vi "N Closest Point.vi"(6 "Index to ignore Array":i32[](array[numeric]), 8 "line index":i32, 9 "Y in":dbl=359.5 format="%#_13g", 10 "X in":dbl=18.050867335505 format="%#_13g", 11 "All Lines":T1) -> (0 "Index on Line":i32, 3 "Array size":i32)   [LabVIEW 2014]
uses:
  Libraries/Map Data Folder/All-Lines.ctl
  Libraries/Map Data Folder/LineCluster.ctl
  Libraries/Map Data Folder/LineConnection.ctl
  Libraries/Map Data Folder/Map Data.lvlib
panel:
  out "Index found?":bool
  out "Distance to nearest":dbl
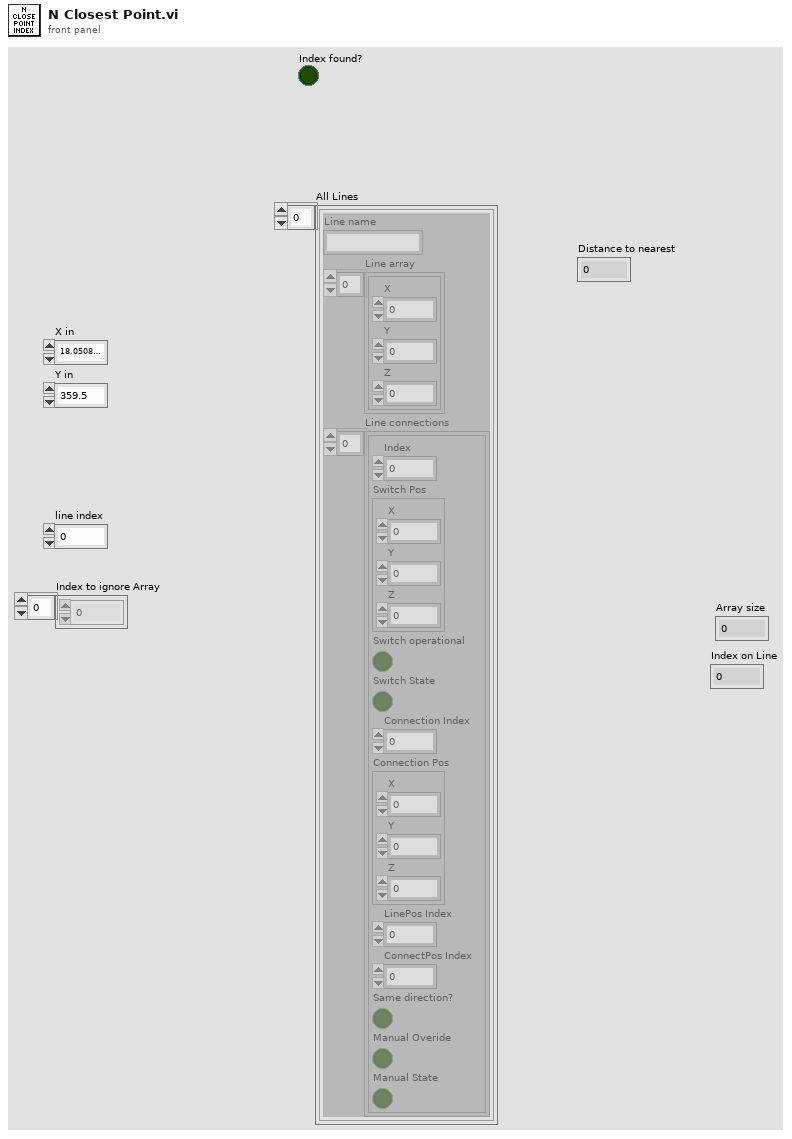
[diagram p1: front panel]
types:
  T1 = typedef "Map Data.lvlib/All-Lines.ctl" = T2[]
  T2 = typedef "Map Data.lvlib/LineCluster.ctl" = cluster{"Line name":string, "Line array":cluster{"X":dbl, "Y":dbl, "Z":dbl}[], "Line connections":T3[]}
  T3 = typedef "Map Data.lvlib/LineConnection.ctl" = cluster{"Index":i32, "Switch Pos":cluster{"X":dbl, "Y":dbl, "Z":dbl}, "Switch operational":bool, "Switch State":bool, "Connection Index":i32, "Connection Pos":cluster{"X":dbl, "Y":dbl, "Z":dbl}, "LinePos Index":i32, "ConnectPos Index":i32, "Same direction?":bool, "Manual Overide":bool, "Manual State":bool}
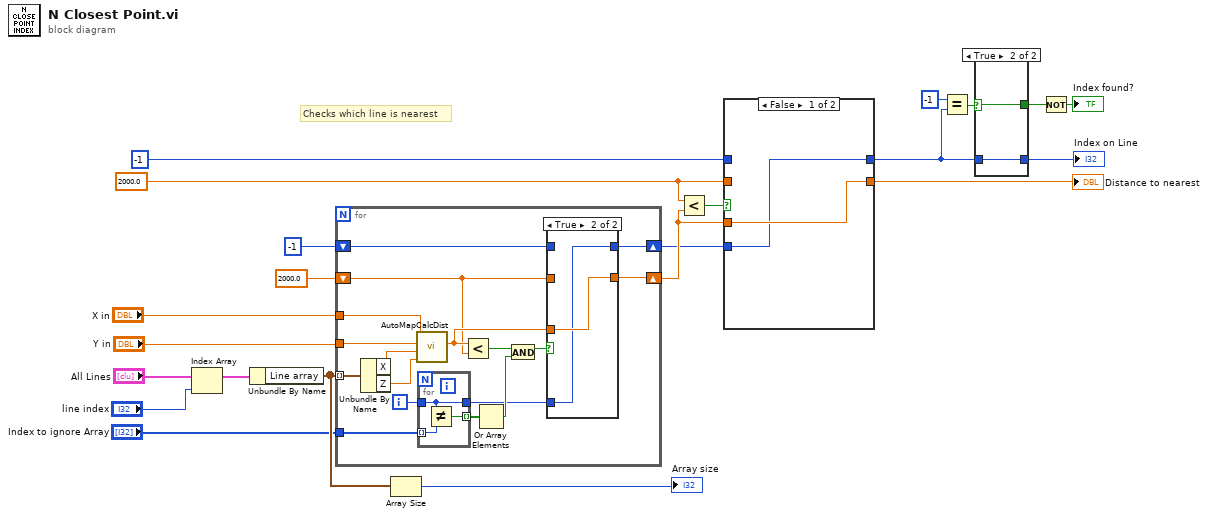
[diagram p0: block diagram]
diagram:
  w21 = 2000.0 ("Distance")
  # "Checks which line is nearest"
  n1 = Index Array(array="All Lines", index="line index") -> (element=w9:T2)
  n2 = Unbundle By Name(w9) -> ("Line array"=w3:cluster{"X":dbl, "Y":dbl, "Z":dbl}[])
  n3 = for {
    tunnel: "X in" -> [w39]
    tunnel: w3 -> [w38] mode=indexing
    tunnel: "Y in" -> [w35]
    shift-right: [w32] -> w13
    shift-left: 2000.0 ("Distance") -> [w33]
    shift-right: [w30] -> w10
    shift-left: -1 -> [w31]
    tunnel: "Index to ignore Array" -> [w27]
    i -> [w28]
    n4 = Unbundle By Name(w38) -> ("X"=w36:dbl, "Z"=w37:dbl)
    n5 = call "AutoMapCalcDist.vi"("Y2"=w37, "X2"=w36, "Y1"=w35, "X1"=w39) -> ("Distance"=w34:dbl)  [unwired: 7 in]
    n6 = for {
      tunnel: w28 -> [w40]
      tunnel: w27 -> [w42] mode=indexing
      tunnel: [w41] -> w25 mode=indexing
      tunnel: [w40] -> w23
      n7 = Not Equal?(x=w40, y=w42) -> (x != y?=w41:bool)
    }
    n8 = Less?(x=w34, y=w33) -> (x < y?=w29:bool)
    n9 = Or Array Elements(Boolean array=w25) -> (logical OR=w24:bool)
    n10 = And(x=w29, y=w24) -> (x .and. y?=w26:bool)
    n11 = case shown="True" w26 {
      tunnel: w34 -> [_ w46]
      tunnel: [w44 w46] -> w32
      tunnel: w33 -> [w44 _]
      tunnel: w31 -> [w43 _]
      tunnel: w23 -> [_ w45]
      tunnel: [w43 w45] -> w30
      frame False {
      }
      frame True {
      }
    }
  }
  n12 = Array Size(array=w3) -> (size(s)=→"Array size":i32)
  n13 = Less?(x=w21, y=w13) -> (x < y?=w12:bool)
  n14 = case shown="False" w12 {
    tunnel: w13 -> [w48 _]
    tunnel: [w48 w50] -> w20
    tunnel: w21 -> [_ w50]
    tunnel: -1 -> [_ w49]
    tunnel: w10 -> [w47 _]
    tunnel: [w47 w49] -> w4
    frame False {
    }
    frame True {
    }
  }
  "Distance to nearest" <- w20
  n15 = Equal?(x=-1, y=w4) -> (x = y?=w15:bool)
  n16 = case shown="True" w15 {
    selector: w15 -> [w51 w54]
    tunnel: [w51 w54] -> w16
    tunnel: w4 -> [w52 w53]
    tunnel: [w52 w53] -> w2
    frame False {
    }
    frame True {
    }
  }
  "Index on Line" <- w2
  n17 = Not(x=w16) -> (.not. x?=→"Index found?":bool)
